vi "Spin Up Shooter.vi"(1 "Execute":bool=TRUE, 2 "Manual Speed":dbl) -> (4 "Done Executing":bool)   [LabVIEW 2011]
uses:
  Globals/Calculated Shooter Speed.vi
  Globals/Jaguar Commands.vi
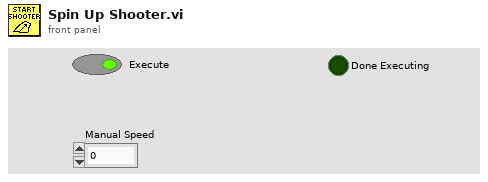
[diagram p1: front panel]
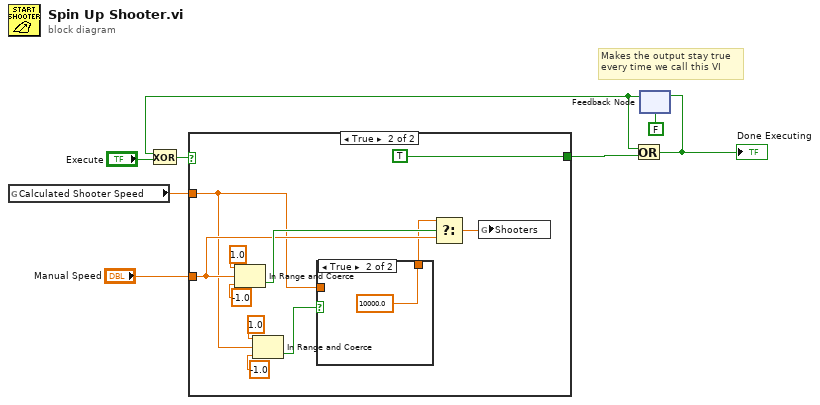
[diagram p0: block diagram]
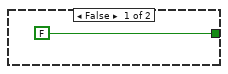
[diagram p2: hidden frame]
diagram:
  # "Makes the output stay true\nevery time we call this VI"
  n1 = global read "Calculated Shooter Speed.vi" "Calculated Shooter Speed"() -> (w1:dbl)
  n2 = feedback #1(FALSE) -> (w4:bool)
  n3 = Exclusive Or(1:"Execute", 2:w4) -> (0:w8:bool)
  n4 = case shown="True" w8 {
    tunnel: [FALSE TRUE] -> w6
    tunnel: "Manual Speed" -> [_ w16]
    tunnel: w1 -> [_ w11]
    frame False {
    }
    frame True {
      n5 = In Range and Coerce(upper limit=1.0, x=w16, lower limit=-1.0) -> (In Range?=w17:bool)  [unwired: 1 out]
      n6 = In Range and Coerce(upper limit=1.0, x=w11, lower limit=-1.0) -> (In Range?=w12:bool)  [unwired: 1 out]
      n7 = case shown="True" w12 {
        tunnel: w11 -> [w21 _]
        tunnel: [w21 10000.0] -> w10
        frame False {
        }
        frame True {
        }
      }
      n8 = Select(t=w10, s=w17, f=w16) -> (s? t:f=w15:dbl)
      n9 = global write "Jaguar Commands.vi" "Shooters"(w15) -> ()
    }
  }
  n10 = Or(x=w4, y=w6) -> (x .or. y?=w3:bool)
  "Done Executing" <- w3
  n11 = feedback-in #1(w3) -> ()
